vi "LcWebView_DoughnutPlot_Example.vi"() -> ()   [LabVIEW 2018, in "LcWebView.lvclass"]
doc: "Inject javascript arguments"
uses:
  LcWebView.lvclass
  D:/GitProjects/Public/GitHub/LcWebView/data/Microsoft.Web.WebView2.WinForms.dll
  data/Microsoft.Web.WebView2.WinForms.dll
  ctrls/PlotType.ctl
  ctrls/PiePlotOption.ctl
  ctrls/GenericPlotOption.ctl
  ctrls/LegendPosition.ctl
  <userlib>/_OpenG.lib/numeric/numeric.llb/Random Number Within Range - DBL__ogtk.vi
panel:
  out "BrowserProcessId":u32
  out "Status Message":string
  in  "stop":bool
  in  "Web":refnum<k24>(container)
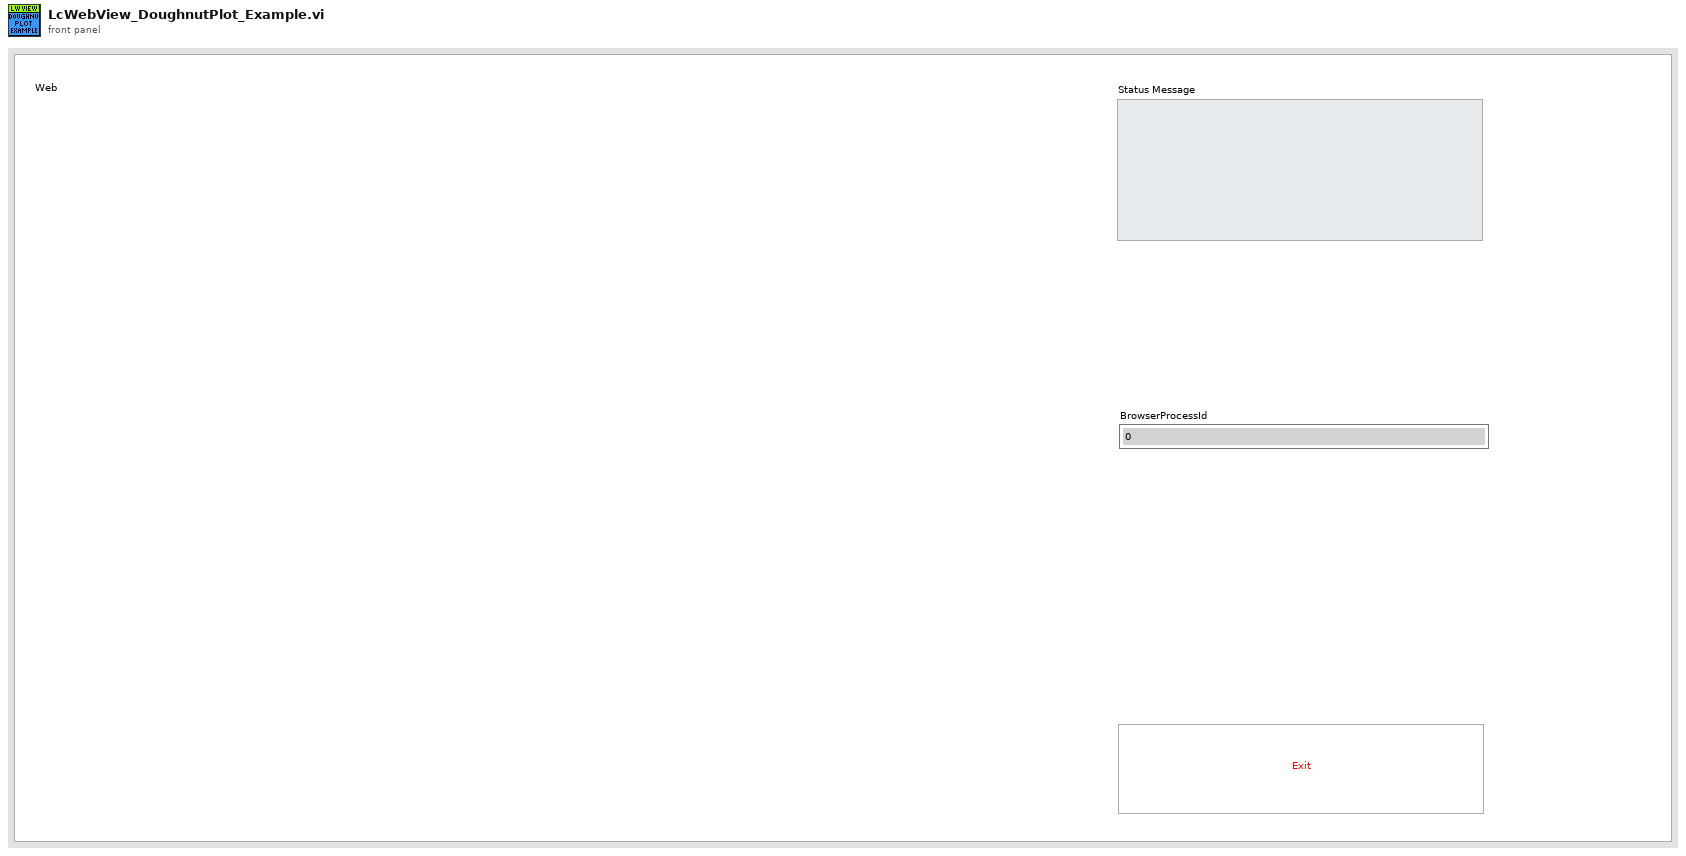
[diagram p1: front panel]
types:
  T1 = typedef "LcWebView.lvclass/GenericPlotOption.ctl" = cluster{"GraphTitle":string, "LegendDisplay":bool, "LegendPosition":T2}
  T2 = typedef "LcWebView.lvclass/LegendPosition.ctl" = enum16{"top", "right", "left", "bottom"}
  T3 = typedef "LcWebView.lvclass/PiePlotOption.ctl" = cluster{"cutoutPercentage":i32}
  T4 = typedef "LcWebView.lvclass/PlotType.ctl" = enum16{"bar", "line", "pie", "doughnut", "scatter", "radar", "bubble", "polarArea"}
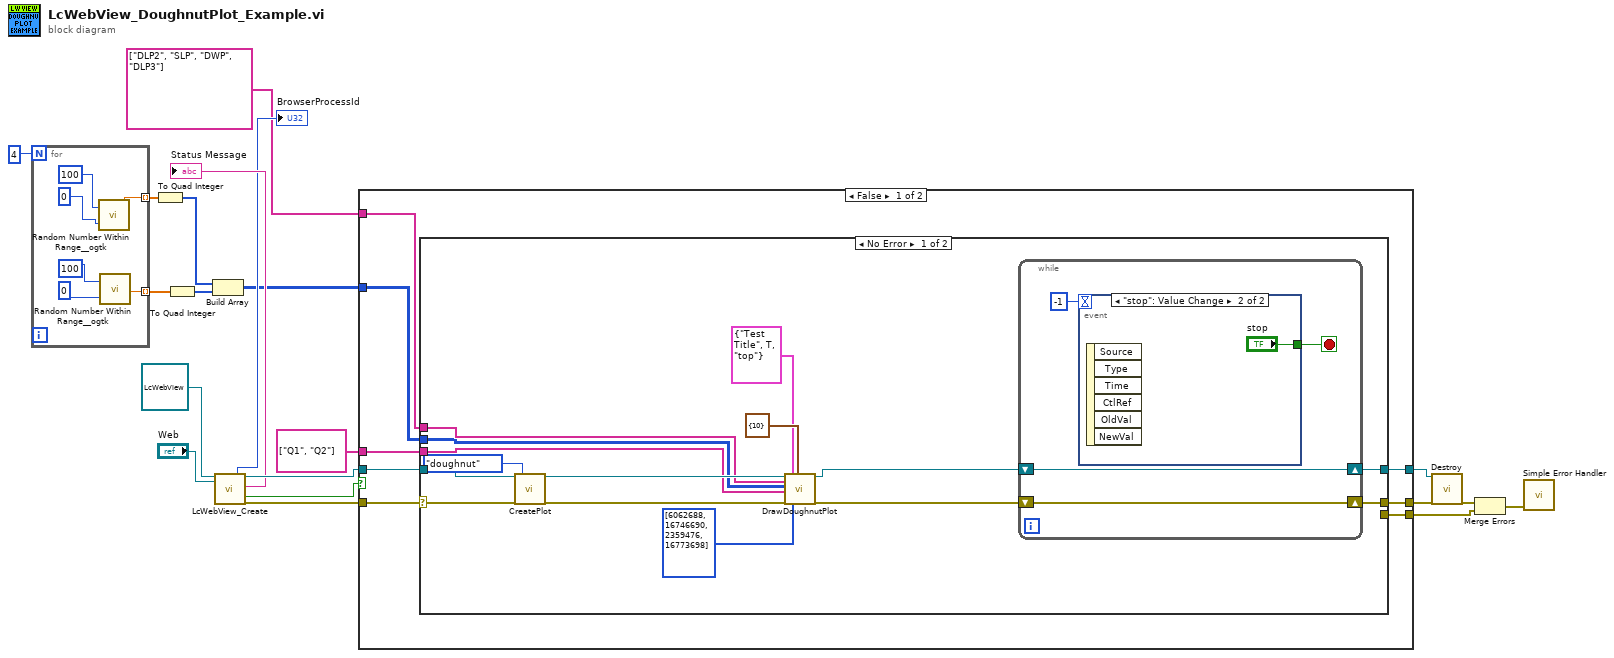
[diagram p0: block diagram]
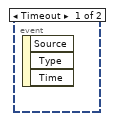
[diagram p2: hidden frame]
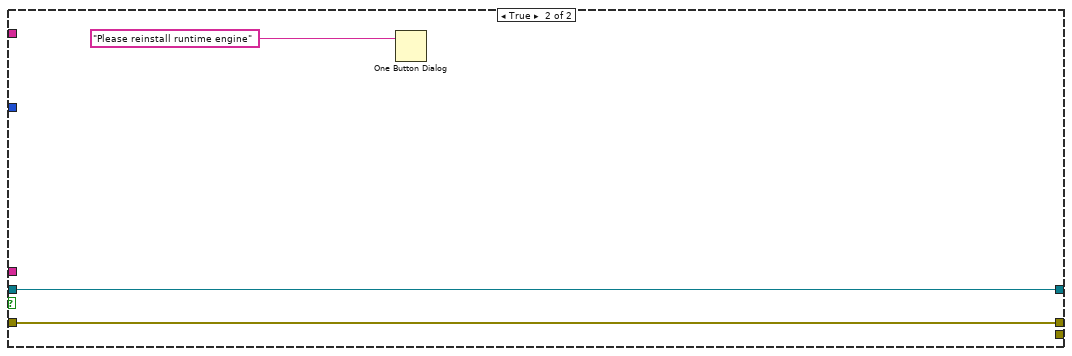
[diagram p4: hidden frame]
diagram:
  n1 = for {
    N: 4 -> [_]
    tunnel: [w24] -> w8 mode=indexing
    tunnel: [w21] -> w9 mode=indexing
    n2 = call-poly <userlib>:"Random Number Within Range__ogtk.vi"("High"=i64 100 ("upper bound (100)"), "Low"=i64 0 ("lower bound (-100)")) -> ("Random Number"=w24:dbl)  [unwired: 3 in]
    n3 = call-poly <userlib>:"Random Number Within Range__ogtk.vi"("High"=i64 100 ("upper bound (100)"), "Low"=i64 0 ("lower bound (-100)")) -> ("Random Number"=w21:dbl)  [unwired: 3 in]
  }
  n4 = To Quad Integer(1:w8) -> (0:w2:i64[])
  n5 = To Quad Integer(1:w9) -> (0:w1:i64[])
  n6 = Build Array(w2, w1) -> (w4:i64[][])
  n7 = call "LcWebView_Create.vi"("reference in"=refnum<class "LcWebView.lvclass"> refnum, "Webview container"="Web") -> ("BrowserProcessId"=→"BrowserProcessId":u32, "reference out"=w18:refnum<class "LcWebView.lvclass">, "Status Message"=→"Status Message":string, "Reinstall Runtime"=w11:bool, "Error Out"=w17:errorcluster)  [unwired: 10 in, 3 out]
  n8 = case shown="False" w11 {
    tunnel: w18 -> [w34 w59]
    tunnel: w17 -> [w33 w58]
    tunnel: [w32 w59] -> w16
    tunnel: [w30 w58] -> w15
    tunnel: [w31 _] -> w12
    tunnel: string[] ["DLP2", "SLP", "DWP", "DLP3"] ("DatasetLabels") -> [w29 _]
    tunnel: string[] ["Q1", "Q2"] ("PiePlot.PlotLabels") -> [w28 _]
    tunnel: w4 -> [w27 _]
    frame False {
      n9 = case shown="No Error" w33 {
        selector: w33 -> [w47 w55]
        tunnel: w34 -> [w48 w56]
        tunnel: [w43 w56] -> w32
        tunnel: [w49 _] -> w30
        tunnel: [_ w55] -> w31
        tunnel: w29 -> [w41 _]
        tunnel: w28 -> [w40 _]
        tunnel: w27 -> [w39 _]
        frame No Error {
          n10 = call-dynamic "CreatePlot.vi"("reference in"=w48, "Error In"=w47, "PlotType"=PlotType."doughnut") -> ("reference out"=w46:refnum<class "LcWebView.lvclass">, "Error Out"=w35:errorcluster)  [unwired: 15 in]
          n11 = call-dynamic "DrawDoughnutPlot.vi"("reference in"=w46, "PiePlot.PlotLabels"=w41, "PiePlot.Dataset"=w39, "PiePlot.DatasetLabels"=w40, "Error In"=w35, "GenericPlotOptions"=T1 {"GraphTitle"="Test Title", "LegendDisplay"=TRUE, "LegendPosition"=enum."top"}, "PiePlot.PlotColours"=u32[] [6062688, 16746690, 2359476, 16773698] ("PlotColours"), "PiePlotOptions"=T3 {"cutoutPercentage"=10}) -> ("reference out"=w44:refnum<class "LcWebView.lvclass">, "Error Out"=w45:errorcluster)  [unwired: 10 in]
          n12 = while {
            shift-right: [w53] -> w43
            shift-left: w44 -> [w53]
            shift-right: [w52] -> w49
            shift-left: w45 -> [w52]
            stop <- w50 stop-if-true
            n13 = event shown="[1] \"stop\": Value Change" {
              selector: _ -> [_ _]
              dyn-events: _ -> [_ _]
              timeout: -1 -> [_ _]
              tunnel: [_ "stop"] -> w50
              event Timeout {
                n14 = event-data() -> ()  [unwired: 1 in, 3 out]
              }
              event "stop": Value Change {
                n15 = event-data() -> ()  [unwired: 1 in, 6 out]
              }
            }
          }
        }
        frame Error {
        }
      }
    }
    frame True {
      n16 = One Button Dialog(message="Please reinstall runtime engine") -> ()  [unwired: 1 in, 1 out]
    }
  }
  n17 = call-dynamic "Destroy.vi"("reference in"=w16, "Error In"=w15) -> ("Error Out"=w14:errorcluster)  [unwired: 16 in, 1 out]
  n18 = Merge Errors(w14, w12) -> (w3:errorcluster)
  n19 = call <vilib>:"Simple Error Handler.vi"("error in (no error)"=w3) -> ()  [unwired: 4 in, 5 out]
